vi "Save to ProjFile.vi"(8 "error in (no error)":errorcluster, 11 "LanguageData in":refnum<class "Project Data.lvclass">) -> (0 "error out":errorcluster, 3 "LanguageData out":refnum<class "Project Data.lvclass">)   [LabVIEW 2013, in "SET Project Data.lvlib" / "Project Data.lvclass"]
uses:
  Project Data.lvclass
  Types/ProjFile_Resources Data.ctl
  Types/ProjFile_Language Entry.ctl
  Types/ProjFile_Resource Entry.ctl
  Types/ProjFile_Project Data.ctl
  Types/ProjFile_Menu Data.ctl
  Types/ProjFile_VI Data.ctl
  Types/ProjFile_GObject Data.ctl
  Project Data.lvclass/Project Data.ctl
  Resource Data Class/Resource Data.lvclass/Resource Data.ctl
  Read Menu Table.vi
  Resource Data Class/Read Languages.vi
  Resource Data Class/Read Resources.vi
  Menu Class/Menu Data.lvclass
  VI Class/VI Data.lvclass
  Resource Data Class/Resource Data.lvclass
  SET Project Data.lvlib
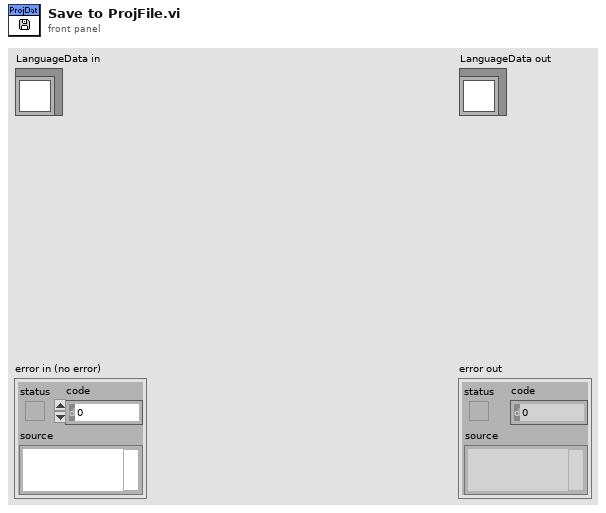
[diagram p1: front panel]
types:
  T1 = typedef "SET Project Data.lvlib/ProjFile_Project Data.ctl" = cluster{"Menu Data[]":T2[], "VI Data[]":T3[]}
  T2 = typedef "SET Project Data.lvlib/ProjFile_Menu Data.ctl" = cluster{"Menu Path":path, "Menu Items[]":cluster{"Tag":string, "RID":string}[]}
  T3 = typedef "SET Project Data.lvlib/ProjFile_VI Data.ctl" = cluster{"VI Path":path, "GObjects[]":T4[]}
  T4 = typedef "SET Project Data.lvlib/ProjFile_GObject Data.ctl" = cluster{"UID":i32, "Label":string, "ClassName":string, "Item List[]":cluster{"Item Name":string, "RID":string}[]}
  T5 = typedef "SET Project Data.lvlib/ProjFile_Resources Data.ctl" = cluster{"Languages []":T6[], "Resources []":T7[]}
  T6 = typedef "SET Project Data.lvlib/ProjFile_Language Entry.ctl" = cluster{"Tag":string, "Name":string, "Code Page":u16}
  T7 = typedef "SET Project Data.lvlib/ProjFile_Resource Entry.ctl" = cluster{"RID":string, "Tag":string, "Strings [] (UTF-16)":string[], "Shared?":bool}
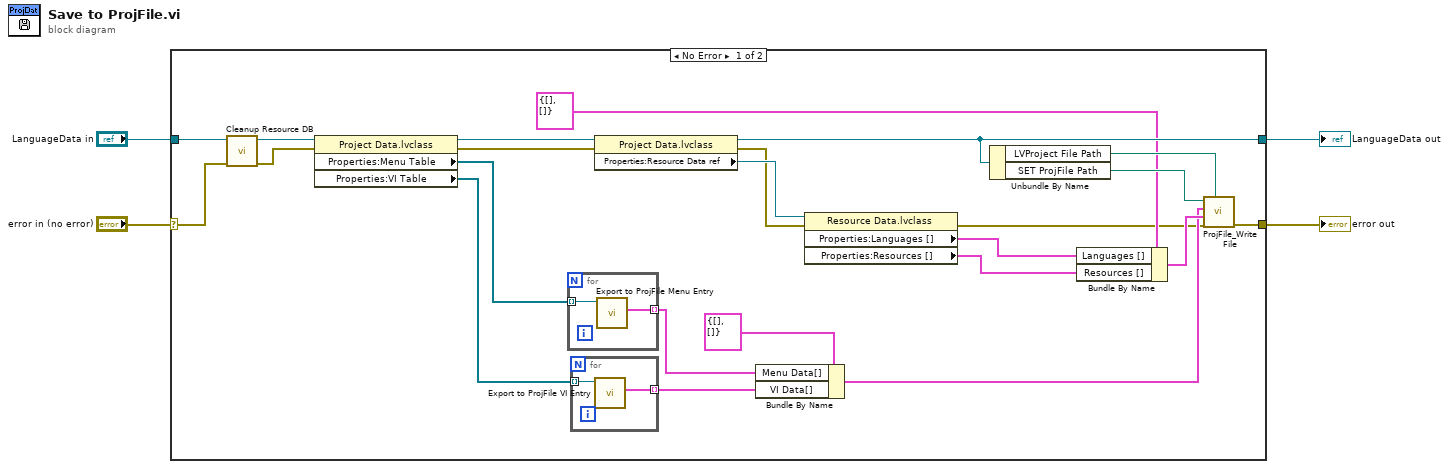
[diagram p0: block diagram]
diagram:
  n1 = case shown="No Error" "error in (no error)" {
    selector: "error in (no error)" -> [w22 w33]
    tunnel: [w26 w33] -> w3
    tunnel: [w17 w32] -> w2
    tunnel: "LanguageData in" -> [w23 w32]
    frame No Error {
      n2 = call-dynamic "Cleanup Resource DB.vi"("error in (no error)"=w22, "ProjectData in"=w23) -> ("error out"=w20:errorcluster, "ProjectData out"=w21:refnum<class "Project Data.lvclass">)  [unwired: 8 in]
      n3 = property class="Project Data.lvclass"(reference=w21, error in=w20) -> (reference out=w19:refnum<class "Project Data.lvclass">, error out=w18:errorcluster, "Properties:Menu Table"=w13:refnum<class "Menu Data.lvclass">[], "Properties:VI Table"=w15:refnum<class "VI Data.lvclass">[])
      n4 = for {
        tunnel: w13 -> [w29] mode=indexing
        tunnel: [w28] -> w12 mode=indexing
        n5 = call "Export to ProjFile Menu Entry.vi"("Menu Data in"=w29) -> ("Menu Data"=w28:T2)  [unwired: 8 in, 2 out]
      }
      n6 = for {
        tunnel: w15 -> [w31] mode=indexing
        tunnel: [w30] -> w14 mode=indexing
        n7 = call "Export to ProjFile VI Entry.vi"("LanguageData in"=w31) -> ("VI Data"=w30:T3)  [unwired: 8 in, 2 out]
      }
      n8 = property class="Project Data.lvclass"(reference=w19, error in=w18) -> (reference out=w17:refnum<class "Project Data.lvclass">, error out=w7:errorcluster, "Properties:Resource Data ref"=w9:refnum<data-value>)
      n9 = Bundle By Name(cluster=T1 {"Menu Data[]"=[], "VI Data[]"=[]} ("Project Data"), "Menu Data[]"=w12, "VI Data[]"=w14) -> (w11:T1)
      n10 = property class="Resource Data.lvclass"(reference=w9, error in=w7) -> (error out=w5:errorcluster, "Properties:Languages []"=w8:T6[], "Properties:Resources []"=w6:T7[])  [unwired: 1 out]
      n11 = Unbundle By Name(w17) -> ("LVProject File Path"=w25:path, "SET ProjFile Path"=w24:path)
      n12 = Bundle By Name(cluster=T5 {"Languages []"=[], "Resources []"=[]} ("Resource Data"), "Languages []"=w8, "Resources []"=w6) -> (w27:T5)
      n13 = call "ProjFile_Write File.vi"("LV Project Path"=w25, "error in"=w5, "Resource Data"=w27, "Project Data"=w11, "file path (use dialog)"=w24) -> ("error out"=w26:errorcluster)  [unwired: 5 in, 1 out]
    }
    frame Error {
    }
  }
  "error out" <- w3
  "LanguageData out" <- w2
